vi "5.4 Acquire Data Voltage.vi"() -> ()   [LabVIEW 2019]
uses:
  <vilib>/DAQmx/read.llb/DAQmx Read (Analog 1D DBL 1Chan NSamp).vi
  <vilib>/DAQmx/miscellaneous.llb/DAQmx Fill In Error Info.vi
  <vilib>/DAQmx/create/channels.llb/DAQmx Create Channel (AI-Voltage-Basic).vi
  <vilib>/DAQmx/configure/timing.llb/DAQmx Timing (Sample Clock).vi
  <resource>/objmgr/daqmx.rc
panel:
  out "Waveform Graph 2":dbl[](graph)
  out "Actual Sample Rate (Hz)":dbl
  in  "Configuration Control":T1={"number of samples"=-1, "Minimum Value"=-1.0, "Maximum Value"=-1.0, "physical channels"="Multi_I-O/ai0", "Desired Sample Rate (Hz)"=-1.0, "sample mode"=10178} {"sample mode" items=["Finite Samples"=10178, "Continuous Samples"=10123, "Hardware Timed Single Point"=12522]}
  out "Waveform Graph":dbl[](graph)
  in  "number of samples per channel":i32=-1
  # "DAQmx Tast"
  # "Full DAQmx API"
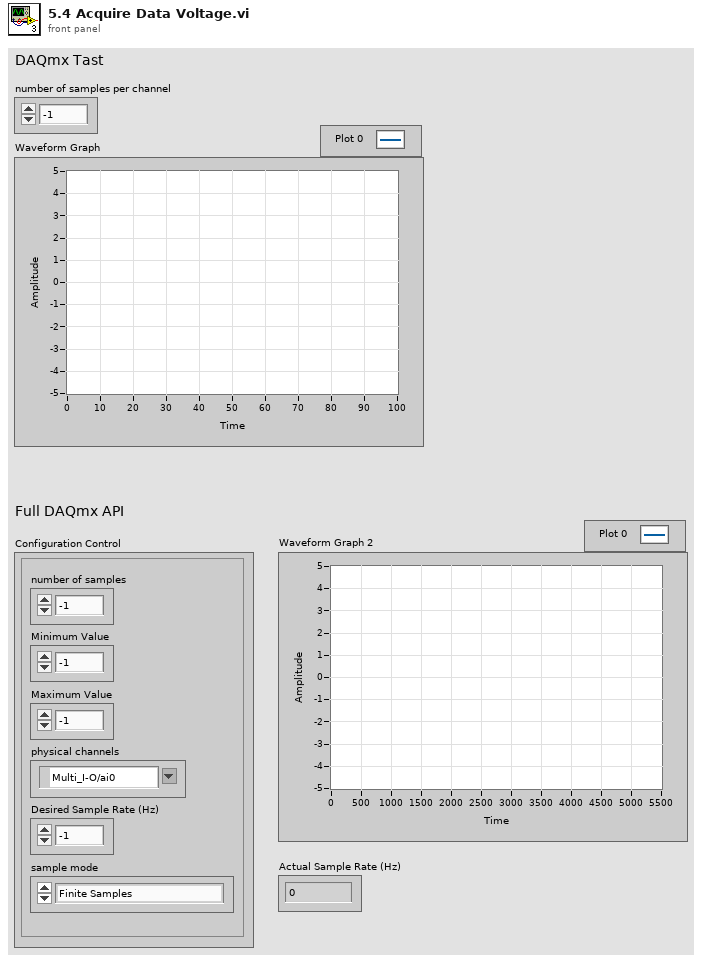
[diagram p1: front panel]
types:
  T1 = cluster{"number of samples":i32, "Minimum Value":dbl, "Maximum Value":dbl, "physical channels":tag, "Desired Sample Rate (Hz)":dbl, "sample mode":i32}
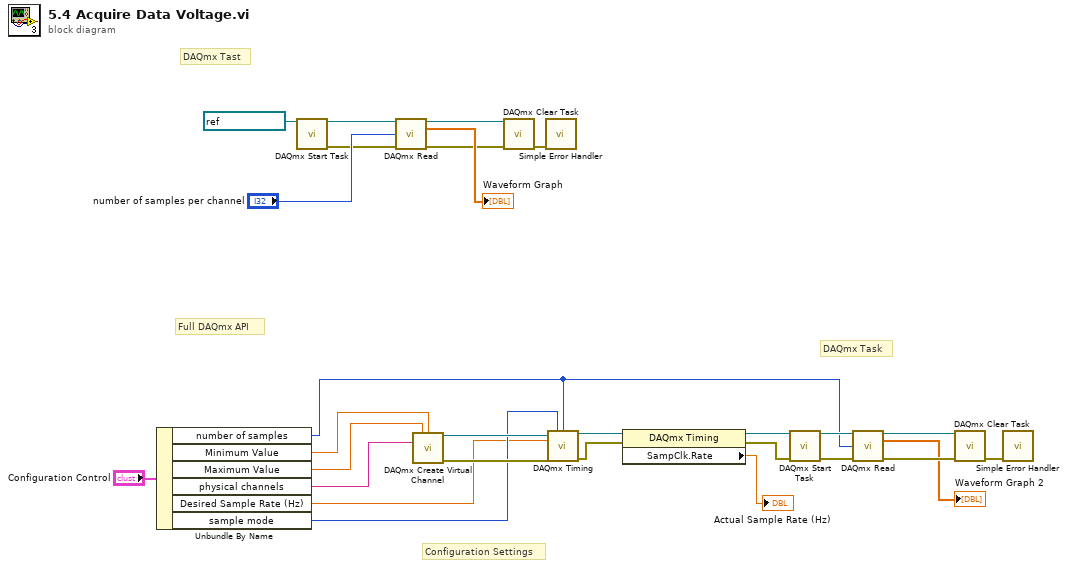
[diagram p0: block diagram]
diagram:
  # "Configuration Settings"
  # "DAQmx Task"
  # "Full DAQmx API"
  # "DAQmx Tast"
  n1 = Unbundle By Name("Configuration Control") -> ("number of samples"=w1:i32, "Minimum Value"=w16:dbl, "Maximum Value"=w17:dbl, "physical channels"=w15:tag, "Desired Sample Rate (Hz)"=w13:dbl, "sample mode"=w14:i32)
  n2 = call <vilib>:"DAQmx Start Task.vi"("task/channels in"=refnum<k21> "AI Voltage") -> ("task out"=w22:refnum<k21>, "error out"=w25:errorcluster)  [unwired: 13 in]
  n3 = call-poly <vilib>:"DAQmx Read.vi"("task/channels in"=w22, "number of samples per channel"="number of samples per channel", "error in"=w25) -> ("task out"=w23:refnum<k21>, "data"=→"Waveform Graph":dbl[], "error out"=w24:errorcluster)  [unwired: 10 in]
  n4 = call-poly <vilib>:"DAQmx Create Virtual Channel.vi"("maximum value"=w17, "minimum value"=w16, "physical channels"=w15) -> ("task out"=w20:refnum<k21>, "error out"=w19:errorcluster)  [unwired: 11 in]
  n5 = call <vilib>:"DAQmx Clear Task.vi"("task in"=w23, "error in"=w24) -> ("error out"=w21:errorcluster)  [unwired: 13 in]
  n6 = call <vilib>:"Simple Error Handler.vi"("error in (no error)"=w21) -> ()  [unwired: 4 in, 5 out]
  n7 = call-poly <vilib>:"DAQmx Timing.vi"("task/channels in"=w20, "sample mode"=w14, "samples per channel"=w1, "rate"=w13, "error in"=w19) -> ("task out"=w11:refnum<k21>, "error out"=w12:errorcluster)  [unwired: 9 in]
  n8 = property class="DAQmx Timing"(reference=w11, error in=w12) -> (reference out=w7:refnum<k21>, error out=w6:errorcluster, "SampClk.Rate"=→"Actual Sample Rate (Hz)":dbl)
  n9 = call <vilib>:"DAQmx Start Task.vi"("task/channels in"=w7, "error in"=w6) -> ("task out"=w9:refnum<k21>, "error out"=w5:errorcluster)  [unwired: 12 in]
  n10 = call-poly <vilib>:"DAQmx Read.vi"("task/channels in"=w9, "number of samples per channel"=w1, "error in"=w5) -> ("task out"=w8:refnum<k21>, "data"=→"Waveform Graph 2":dbl[], "error out"=w4:errorcluster)  [unwired: 10 in]
  n11 = call <vilib>:"DAQmx Clear Task.vi"("task in"=w8, "error in"=w4) -> ("error out"=w3:errorcluster)  [unwired: 13 in]
  n12 = call <vilib>:"Simple Error Handler.vi"("error in (no error)"=w3) -> ()  [unwired: 4 in, 5 out]
